vi "_get_parameters.vi"(8 "error in (no error)":errorcluster, 11 "UV-VIS_AVANTES in":refnum<class "UV-VIS_AVANTES.lvclass">) -> (0 "error out":errorcluster, 2 "DeviceParam":u8[](array[numeric]), 3 "UV-VIS_AVANTES out":refnum<class "UV-VIS_AVANTES.lvclass">)   [LabVIEW 2020, in "UV-VIS_AVANTES.lvclass"]
uses:
  UV-VIS_AVANTES.lvclass
  C:/Dev/TRANCON/Classes/Detector/Detector.lvclass
  Detector.lvclass/Detector.ctl
  UV-VIS_AVANTES.lvclass/UV-VIS_AVANTES.ctl
  Detector.lvclass
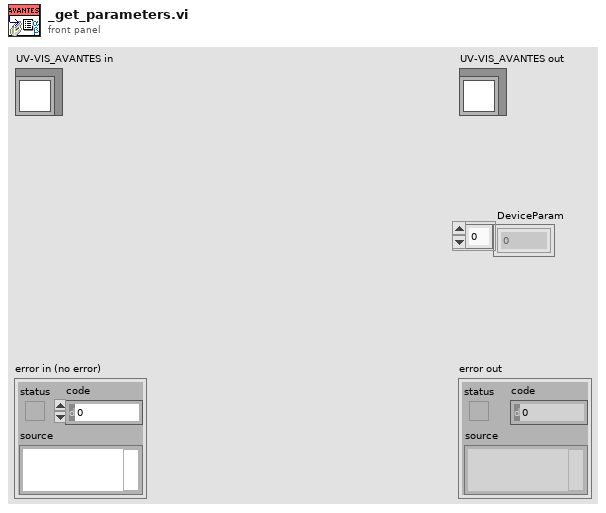
[diagram p1: front panel]
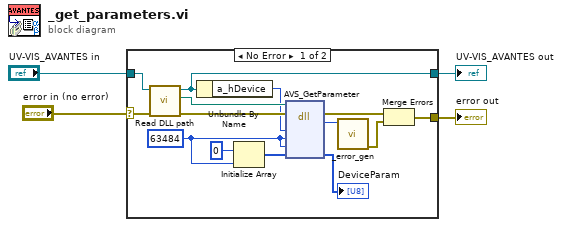
[diagram p0: block diagram]
diagram:
  n1 = case shown="No Error" "error in (no error)" {
    selector: "error in (no error)" -> [w17 w20]
    tunnel: [w5 w20] -> w3
    tunnel: [w11 w19] -> w1
    tunnel: "UV-VIS_AVANTES in" -> [w18 w19]
    frame No Error {
      w12 = u16 63484 ("a_pNumPixelsInput")
      n2 = call "Read DLL path.vi"("error in (no error)"=w17, "Detector in"=w18) -> ("error out"=w15:errorcluster, "DLL path"=w16:path, "Detector out"=w11:refnum<class "UV-VIS_AVANTES.lvclass">)  [unwired: 7 in]
      n3 = Unbundle By Name(w11) -> ("a_hDevice"=w10:i32)
      n4 = Initialize Array(u8 0, w12) -> (w13:u8[])
      n5 = dll-call lib="C:/AvaSpecX64-DLL_9.4/examples/LabView/LabViewSingleChan/avaspec.dll" fn="AVS_GetParameter"(path in=w16, error in=w15, "a_hDevice"=w10, "a_Size"=w12, "a_pRequiredSize"=w12, "a_pDeviceParm"=w13) -> (error out=w7:errorcluster, "return type"=w8:i32, "a_pDeviceParm"=→"DeviceParam":u8[])  [unwired: 4 in, 1 out]
      n6 = call "_error_gen.vi"("return type"=w8) -> ("error out"=w6:errorcluster)  [unwired: 10 in]
      n7 = Merge Errors(w7, w6) -> (w5:errorcluster)
    }
    frame Error {
    }
  }
  "error out" <- w3
  "UV-VIS_AVANTES out" <- w1
